vi "RegisterFile.vi"() -> ()   [LabVIEW 2021]
uses:
  <userlib>/SciSDK/SciSDK_Labview.lvlib
panel:
  out "Register Value Out":i32
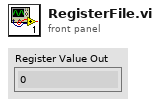
[diagram p1: front panel]
types:
  T1 = cluster{"Name":string, "Board Model":string, "Handle":u64}
  T2 = cluster{"Board Name":string, "Board Model":string, "Handle":u64}
  T3 = cluster{"Register File Path":string, "Register File Name":string}
  T4 = cluster{"Board Name":string, "Board Model":string}
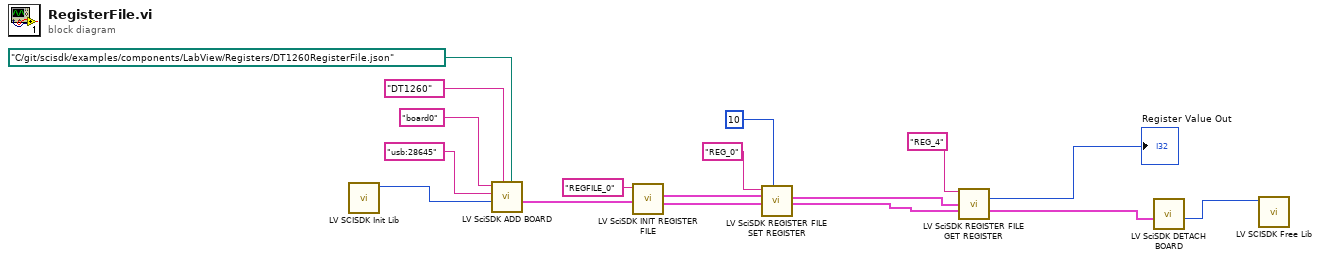
[diagram p0: block diagram]
diagram:
  n1 = call <userlib>:"LV SCISDK Init Lib.vi"() -> ("function return"=w17:u64)  [unwired: 11 in]
  n2 = call <userlib>:"LV SciSDK ADD BOARD.vi"("JsonFile"=path "C:/git/scisdk/examples/components/LabView/Registers/DT1260RegisterFile.json", "Board Model"="DT1260", "SciSDK Handle"=w17, "DevicePath"="usb:28645", "Name"="board0") -> ("Board Handle Out"=w12:T1)  [unwired: 4 in, 2 out]
  n3 = call <userlib>:"LV SciSDK INIT REGISTER FILE.vi"("Handle In"=w12, "Register file name"="REGFILE_0") -> ("Handle Out"=w10:T2, "Register File Handle Out"=w9:T3)  [unwired: 8 in]
  n4 = call <userlib>:"LV SciSDK REGISTER FILE SET REGISTER.vi"("Value"=10, "Board Handle In"=w10, "Register File Handle In"=w9, "Register Name"="REG_0") -> ("Board Handle Out"=w3:T2, "Register File Handle Out"=w4:T4)  [unwired: 4 in, 2 out]
  n5 = call <userlib>:"LV SciSDK REGISTER FILE GET REGISTER.vi"("Register Name"="REG_4", "Register File Handle In"=w4, "Board Handle In"=w3) -> ("Register Value Out"=→"Register Value Out":i32, "Board Handle Out"=w1:T2)  [unwired: 8 in, 3 out]
  n6 = call <userlib>:"LV SciSDK DETACH BOARD.vi"("Board Handle In"=w1) -> ("SciSDK Handle"=w2:u64)  [unwired: 9 in, 1 out]
  n7 = call <userlib>:"LV SCISDK Free Lib.vi"("handle"=w2) -> ()  [unwired: 9 in, 2 out]
